vi "Close.vi"(6 "ACK":bool, 8 "error in":errorcluster) -> (0 "error out":errorcluster, 3 "Response":string)   [LabVIEW 2015, in "Generic Module Library.lvlib" / "Template G_Module.lvlib"]
uses:
  Template G_Module.lvlib
  Private Controls/Module Message Cluster Components/Message Data Cluster.ctl
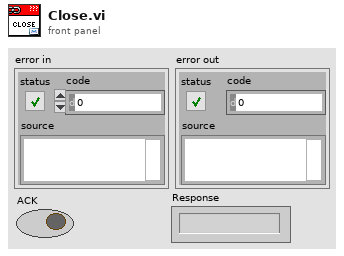
[diagram p1: front panel]
types:
  T1 = typedef "Generic Module Library.lvlib/Template G_Module.lvlib/Message Data Cluster.ctl" = cluster{"Module Action":string, "Message Data":variant}
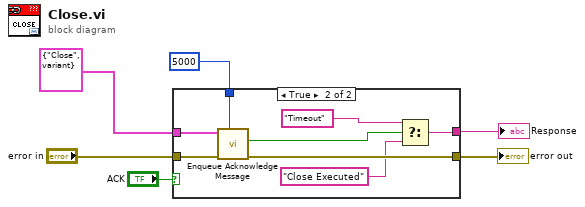
[diagram p0: block diagram]
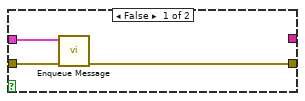
[diagram p2: hidden frame]
diagram:
  n1 = case shown="True" "ACK" {
    tunnel: "error in" -> [w9 w16]
    tunnel: [w8 w17] -> w5
    tunnel: T1 {"Module Action"="Close", "Message Data"=variant} ("Message Data") -> [w7 w15]
    tunnel: 5000 ("Ack Timeout") -> [_ w14]
    tunnel: [_ w11] -> w1
    frame False {
      n2 = call "Enqueue Message.vi"("error in"=w9, "Message Data"=w7) -> ("error out"=w8:errorcluster)  [unwired: 9 in]
    }
    frame True {
      n3 = call "Enqueue Acknowledge Message.vi"("Ack Timeout"=w14, "error in"=w16, "Message Data"=w15) -> ("error out"=w17:errorcluster, "Timed Out"=w10:bool)  [unwired: 6 in, 1 out]
      n4 = Select(t="Timeout", s=w10, f="Close Executed") -> (s? t:f=w11:string)
    }
  }
  "error out" <- w5
  "Response" <- w1
